vi "compare ctls.vi"() -> ()   [LabVIEW 2012]
uses:
  _ResManager_v86/ID_Resource info.ctl
  _ResManager_v86/IDCloneResMgr.lvlib
panel:
  out "Type":u32[](array[numeric]) format="%.0x"
  out "resources":T1[](array[typedef]) {"type" format="%.0x"}
  out "resources2":T1[](array[typedef]) {"type" format="%.0x"}
  out "Array 2":string[](array[string])
  out "Array":bool[](array[boolean])
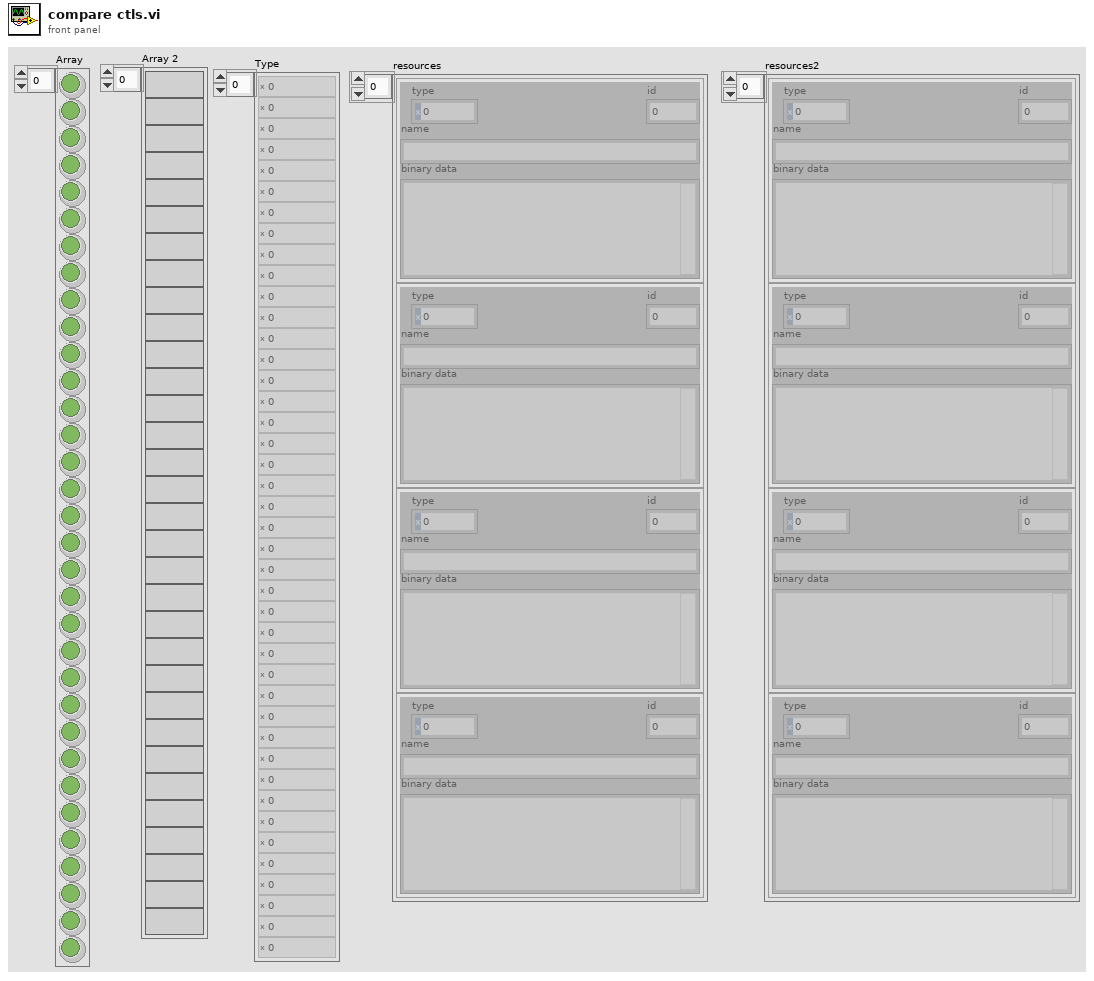
[diagram p1: front panel]
types:
  T1 = typedef "IDCloneResMgr.lvlib/ID_Resource info.ctl" = cluster{"type":u32, "id":i32, "name":string, "binary data":string}
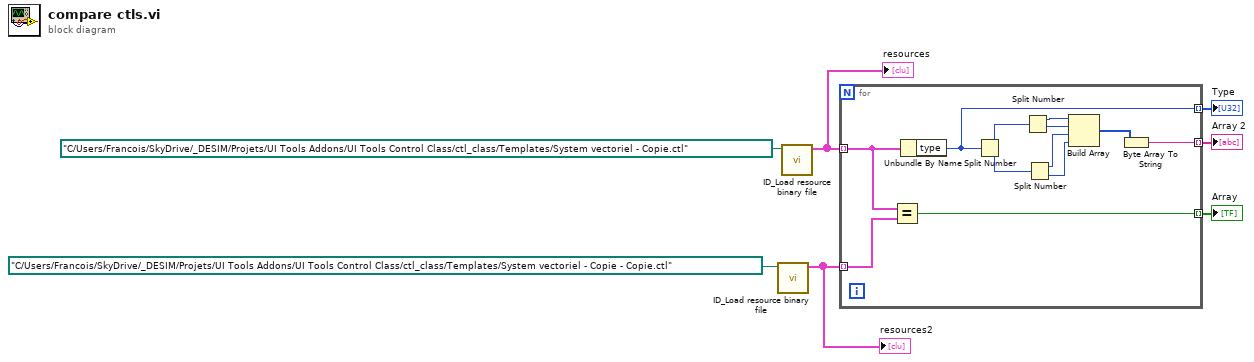
[diagram p0: block diagram]
diagram:
  n1 = call "ID_Load resource binary file.vi"("resource binary file"=path "C:/Users/Francois/SkyDrive/_DESIM/Projets/UI Tools Addons/UI Tools Control Class/ctl_class/Templates/System vectoriel - Copie - Copie.ctl") -> ("resources"=w4:T1[])  [unwired: 8 in, 2 out]
  "resources2" <- w4
  n2 = call "ID_Load resource binary file.vi"("resource binary file"=path "C:/Users/Francois/SkyDrive/_DESIM/Projets/UI Tools Addons/UI Tools Control Class/ctl_class/Templates/System vectoriel - Copie.ctl") -> ("resources"=w5:T1[])  [unwired: 8 in, 2 out]
  "resources" <- w5
  n3 = for {
    tunnel: w5 -> [w17] mode=indexing
    tunnel: w4 -> [w19] mode=indexing
    tunnel: [w18] -> w3 mode=indexing
    tunnel: [w9] -> w2 mode=indexing
    tunnel: [w8] -> w1 mode=indexing
    n4 = Equal?(x=w17, y=w19) -> (x = y?=w18:bool)
    n5 = Unbundle By Name(w17) -> ("type"=w8:u32)
    n6 = Split Number(x=w8) -> (hi(x)=w15:u16, lo(x)=w16:u16)
    n7 = Split Number(x=w15) -> (hi(x)=w14:u8, lo(x)=w13:u8)
    n8 = Split Number(x=w16) -> (hi(x)=w12:u8, lo(x)=w11:u8)
    n9 = Build Array(w14, w13, w12, w11) -> (w10:u8[])
    n10 = Byte Array To String(unsigned byte array=w10) -> (string=w9:string)
  }
  "Array" <- w3
  "Array 2" <- w2
  "Type" <- w1
